vi "ep_Check One Trigger 1pt.vi"(6 "trig. local in":T1, 7 "prev. state in":i8, 8 "error in (no error)":errorcluster, 9 "data time stamp":timestamp, 10 "value in":dbl, 11 "trigger definition":T3) -> (0 "error out":errorcluster, 3 "triggers list":T2(array[cluster]), 4 "trig. local out":T1, 5 "state out":i8)   [LabVIEW 2011, in "NI_EP_Power Quality.lvlib"]
uses:
  <vilib>/addons/Electrical Power/PQ/NI_EP_Power Quality.lvlib
  <vilib>/addons/Electrical Power/PQ/Triggers/subVIs/ep_Trigger Definition.ctl
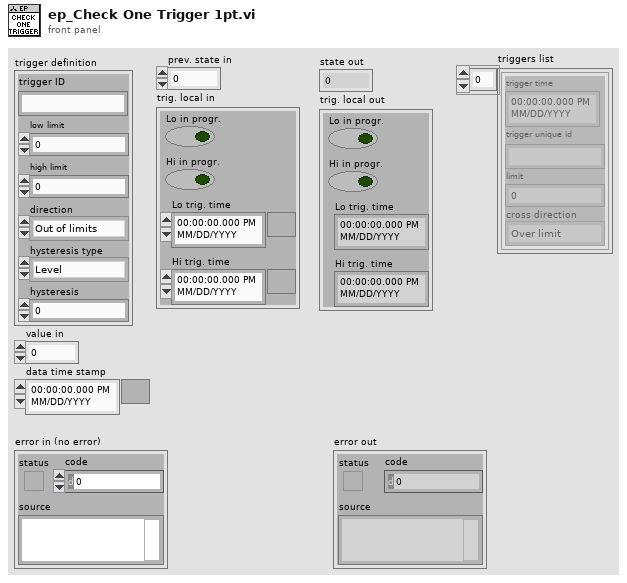
[diagram p1: front panel]
types:
  T1 = cluster{"Lo in progr.":bool, "Hi in progr.":bool, "Lo trig. time":timestamp, "Hi trig. time":timestamp}
  T2 = cluster{"trigger time":timestamp, "trigger unique id":string, "limit":dbl, "cross direction":enum16{"Over limit", "Below limit"}}[]
  T3 = typedef "NI_EP_Power Quality.lvlib/ep_Trigger Definition.ctl" = cluster{"trigger ID":string, "low limit":dbl, "high limit":dbl, "direction":enum16{"Out of limits", "Back to limits", "Both"}, "hysteresis type":enum16{"Level", "Time"}, "hysteresis":dbl}
  T4 = enum16{"Out of limits", "Back to limits", "Both"}
  T5 = cluster{"trigger time":timestamp, "trigger unique id":string, "limit":dbl, "cross direction":enum16{"Over limit", "Below limit"}}
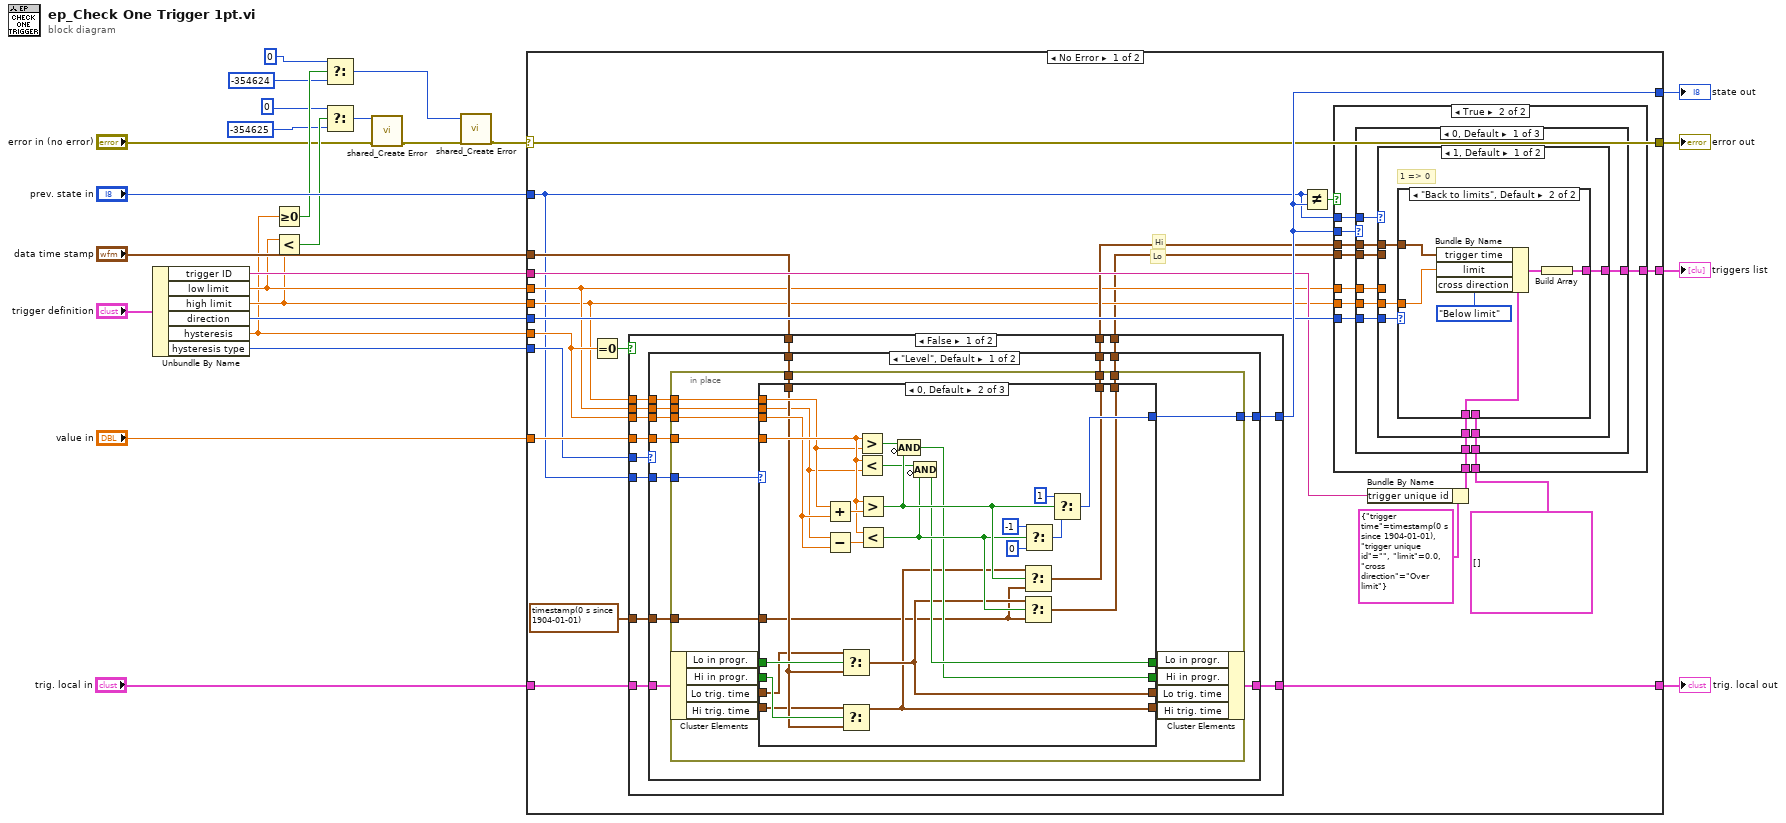
[diagram p0: block diagram]
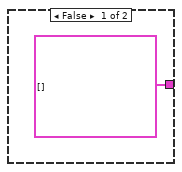
[diagram p2: hidden frame]
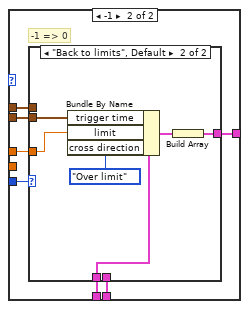
[diagram p4: hidden frame]
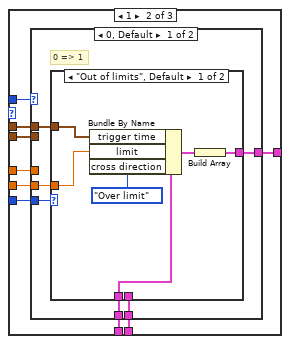
[diagram p6: hidden frame]
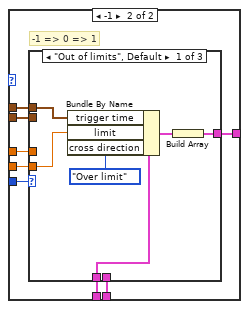
[diagram p8: hidden frame]
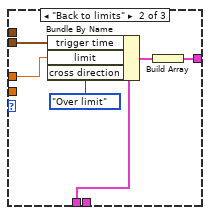
[diagram p9: hidden frame]
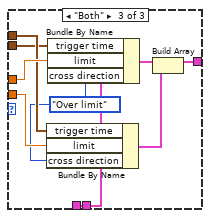
[diagram p10: hidden frame]
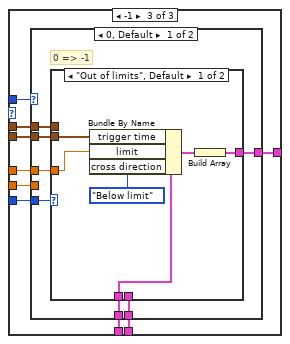
[diagram p11: hidden frame]
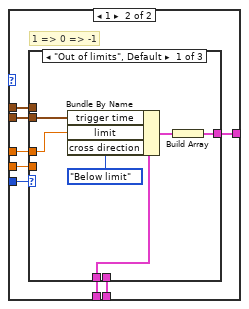
[diagram p13: hidden frame]
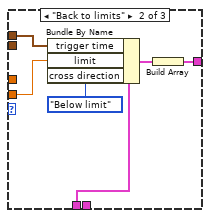
[diagram p14: hidden frame]
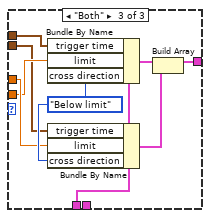
[diagram p15: hidden frame]
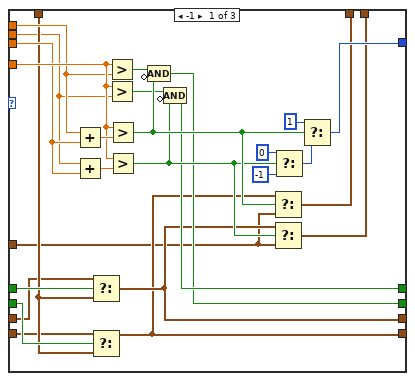
[diagram p16: hidden frame]
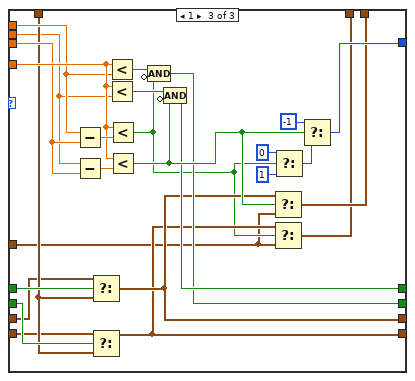
[diagram p17: hidden frame]
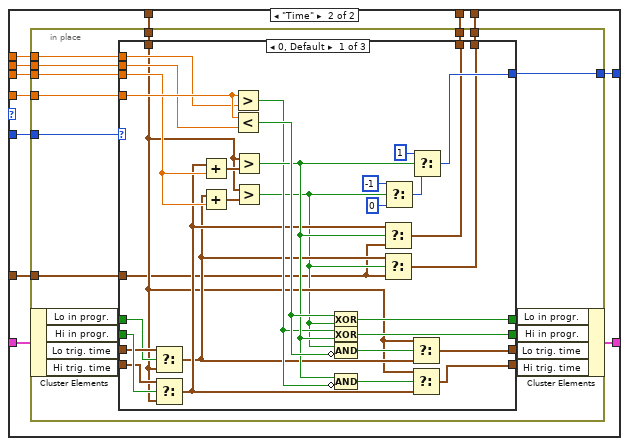
[diagram p18: hidden frame]
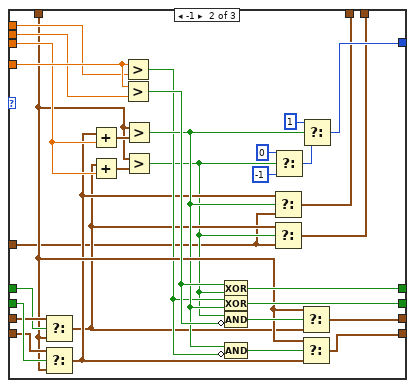
[diagram p19: hidden frame]
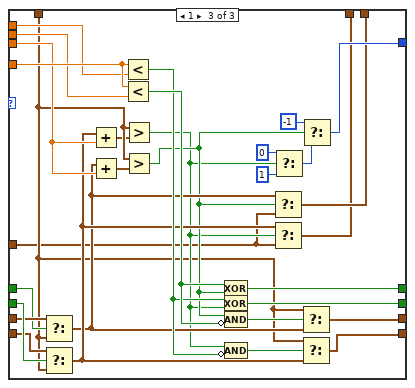
[diagram p20: hidden frame]
diagram:
  n1 = Unbundle By Name("trigger definition") -> ("trigger ID"=w22:string, "low limit"=w15:dbl, "high limit"=w14:dbl, "direction"=w23:T4, "hysteresis"=w11:dbl, "hysteresis type"=w16:enum16{"Level", "Time"})
  n2 = Greater Or Equal To 0?(x=w11) -> (x >= 0?=w10:bool)
  n3 = Less?(x=w15, y=w14) -> (x < y?=w13:bool)
  n4 = Select(t=0 ("error code (0)"), s=w10, f=-354624 ("error code (0)")) -> (s? t:f=w5:i32)
  n5 = Select(t=0 ("error code (0)"), s=w13, f=-354625 ("error code (0)")) -> (s? t:f=w1:i32)
  n6 = call <vilib>:"shared_Create Error.vi"("error in (no error)"="error in (no error)", "error code (0)"=w1) -> ("error out"=w3:errorcluster)  [unwired: 9 in]
  n7 = call <vilib>:"shared_Create Error.vi"("error in (no error)"=w3, "error code (0)"=w5) -> ("error out"=w6:errorcluster)  [unwired: 9 in]
  n8 = case shown="No Error" w6 {
    selector: w6 -> [w29 w460]
    tunnel: "value in" -> [w47 _]
    tunnel: [w45 _] -> w24
    tunnel: w23 -> [w44 _]
    tunnel: w22 -> [w42 _]
    tunnel: [w40 _] -> w21
    tunnel: w11 -> [w38 _]
    tunnel: [w37 _] -> w20
    tunnel: "prev. state in" -> [w28 _]
    tunnel: "data time stamp" -> [w36 _]
    tunnel: "trig. local in" -> [w34 _]
    tunnel: w16 -> [w32 _]
    tunnel: w15 -> [w31 _]
    tunnel: w14 -> [w30 _]
    tunnel: [w29 w460] -> w12
    frame No Error {
      # "Lo"
      # "Hi"
      n9 = Equal To 0?(x=w38) -> (x = 0?=w48:bool)
      n10 = case shown="False" w48 {
        tunnel: w47 -> [w203 w448]
        tunnel: w30 -> [w206 w450]
        tunnel: w31 -> [w205 w449]
        tunnel: [w210 w451] -> w45
        tunnel: w32 -> [w211 _]
        tunnel: w38 -> [w204 _]
        tunnel: w34 -> [w209 w447]
        tunnel: [w208 w447] -> w37
        tunnel: w28 -> [w207 _]
        tunnel: w36 -> [w202 w446]
        tunnel: [w201 w446] -> w35
        tunnel: timestamp(0 s since 1904-01-01) ("f") -> [w200 _]
        tunnel: [w199 w446] -> w27
        frame False {
          n11 = case shown="\"Level\", Default" w211 {
            tunnel: [w213 w330] -> w210
            tunnel: w209 -> [w222 w334]
            tunnel: [w221 w324] -> w208
            tunnel: w207 -> [w215 w329]
            tunnel: w206 -> [w219 w325]
            tunnel: w205 -> [w218 w326]
            tunnel: w204 -> [w217 w327]
            tunnel: w203 -> [w216 w328]
            tunnel: w202 -> [w220 w332]
            tunnel: [w214 w331] -> w201
            tunnel: w200 -> [w223 w333]
            tunnel: [w212 w323] -> w199
            frame "Level", Default {
              n12 = in-place {
                in-place-border: w223 -> [w233]
                in-place-border: w220 -> [w232]
                in-place-border: w219 -> [w231]
                in-place-border: w218 -> [w230]
                in-place-border: w217 -> [w229]
                in-place-border: w216 -> [w228]
                in-place-border: w215 -> [w227]
                in-place-border: [w226] -> w214
                in-place-border: [w225] -> w213
                in-place-border: [w224] -> w212
                n13 = in-place-cluster #1(w222) -> ("Lo in progr."=w241:bool, "Hi in progr."=w240:bool, "Lo trig. time"=w239:timestamp, "Hi trig. time"=w238:timestamp)
                n14 = case shown="0, Default" w227 {
                  tunnel: w241 -> [w253 w280 w310]
                  tunnel: w240 -> [w252 w279 w309]
                  tunnel: w239 -> [w249 w276 w304]
                  tunnel: w238 -> [w248 w275 w305]
                  tunnel: w231 -> [w266 w293 w320]
                  tunnel: w230 -> [w250 w277 w307]
                  tunnel: w229 -> [w265 w292 w319]
                  tunnel: w228 -> [w267 w294 w321]
                  tunnel: w232 -> [w251 w278 w308]
                  tunnel: [w259 w286 w313] -> w225
                  tunnel: [w258 w285 w296] -> w226
                  tunnel: w233 -> [w242 w270 w297]
                  tunnel: [w247 w274 w303] -> w237
                  tunnel: [w246 w273 w302] -> w236
                  tunnel: [w245 w272 w301] -> w235
                  tunnel: [w244 w271 w300] -> w234
                  tunnel: [w243 w269 w298] -> w224
                  frame -1 {
                    n15 = Add(x=w266, y=w265) -> (x+y=w268:dbl)
                    n16 = Add(x=w250, y=w265) -> (x+y=w264:dbl)
                    n17 = Select(t=w249, s=w253, f=w251) -> (s? t:f=w245:timestamp)
                    n18 = Select(t=w248, s=w252, f=w251) -> (s? t:f=w244:timestamp)
                    n19 = Greater?(x=w267, y=w266) -> (0:w257:bool)
                    n20 = Greater?(x=w267, y=w250) -> (0:w255:bool)
                    n21 = Greater?(x=w267, y=w268) -> (0:w256:bool)
                    n22 = Greater?(x=w267, y=w264) -> (0:w254:bool)
                    n23 = Compound Arithmetic op=AND(w257, invert w256) -> (w246:bool)
                    n24 = Compound Arithmetic op=AND(w255, invert w254) -> (w247:bool)
                    n25 = Select(t=w244, s=w256, f=w242) -> (s? t:f=w258:timestamp)
                    n26 = Select(t=w245, s=w254, f=w242) -> (s? t:f=w243:timestamp)
                    n27 = Select(t=i8 0 ("f"), s=w254, f=i8 -1) -> (s? t:f=w261:i8)
                    n28 = Select(t=i8 1 ("f"), s=w256, f=w261) -> (s? t:f=w259:i8)
                  }
                  frame 0, Default {
                    n29 = Add(x=w293, y=w292) -> (x+y=w295:dbl)
                    n30 = Subtract(x=w277, y=w292) -> (x-y=w291:dbl)
                    n31 = Select(t=w276, s=w280, f=w278) -> (s? t:f=w272:timestamp)
                    n32 = Select(t=w275, s=w279, f=w278) -> (s? t:f=w271:timestamp)
                    n33 = Greater?(x=w294, y=w293) -> (0:w284:bool)
                    n34 = Less?(x=w294, y=w277) -> (x < y?=w282:bool)
                    n35 = Greater?(x=w294, y=w295) -> (0:w283:bool)
                    n36 = Less?(x=w294, y=w291) -> (x < y?=w281:bool)
                    n37 = Compound Arithmetic op=AND(w284, invert w283) -> (w273:bool)
                    n38 = Compound Arithmetic op=AND(w282, invert w281) -> (w274:bool)
                    n39 = Select(t=w271, s=w283, f=w270) -> (s? t:f=w285:timestamp)
                    n40 = Select(t=w272, s=w281, f=w270) -> (s? t:f=w269:timestamp)
                    n41 = Select(t=i8 -1 ("f"), s=w281, f=i8 0) -> (s? t:f=w288:i8)
                    n42 = Select(t=i8 1 ("f"), s=w283, f=w288) -> (s? t:f=w286:i8)
                  }
                  frame 1 {
                    n43 = Subtract(x=w320, y=w319) -> (x-y=w322:dbl)
                    n44 = Subtract(x=w307, y=w319) -> (x-y=w318:dbl)
                    n45 = Select(t=w304, s=w310, f=w308) -> (s? t:f=w301:timestamp)
                    n46 = Select(t=w305, s=w309, f=w308) -> (s? t:f=w300:timestamp)
                    n47 = Less?(x=w321, y=w320) -> (x < y?=w312:bool)
                    n48 = Less?(x=w321, y=w307) -> (x < y?=w311:bool)
                    n49 = Less?(x=w321, y=w322) -> (x < y?=w299:bool)
                    n50 = Less?(x=w321, y=w318) -> (x < y?=w306:bool)
                    n51 = Compound Arithmetic op=AND(w312, invert w299) -> (w302:bool)
                    n52 = Compound Arithmetic op=AND(w311, invert w306) -> (w303:bool)
                    n53 = Select(t=w301, s=w306, f=w297) -> (s? t:f=w298:timestamp)
                    n54 = Select(t=w300, s=w299, f=w297) -> (s? t:f=w296:timestamp)
                    n55 = Select(t=i8 0 ("f"), s=w299, f=i8 1) -> (s? t:f=w315:i8)
                    n56 = Select(t=i8 -1 ("f"), s=w306, f=w315) -> (s? t:f=w313:i8)
                  }
                }
                n57 = in-place-cluster #1("Lo in progr."=w237, "Hi in progr."=w236, "Lo trig. time"=w235, "Hi trig. time"=w234) -> (w221:T1)
              }
            }
            frame "Time" {
              n58 = in-place {
                in-place-border: w333 -> [w344]
                in-place-border: w332 -> [w343]
                in-place-border: [w342] -> w331
                in-place-border: [w341] -> w330
                in-place-border: w329 -> [w340]
                in-place-border: w328 -> [w339]
                in-place-border: w327 -> [w338]
                in-place-border: w326 -> [w337]
                in-place-border: w325 -> [w336]
                in-place-border: [w335] -> w323
                n59 = in-place-cluster #2(w334) -> ("Lo in progr."=w352:bool, "Hi in progr."=w351:bool, "Lo trig. time"=w350:timestamp, "Hi trig. time"=w349:timestamp)
                n60 = case shown="0, Default" w340 {
                  tunnel: w352 -> [w368 w398 w431]
                  tunnel: w351 -> [w374 w404 w437]
                  tunnel: w350 -> [w372 w402 w435]
                  tunnel: w349 -> [w371 w401 w434]
                  tunnel: w336 -> [w381 w412 w444]
                  tunnel: w337 -> [w373 w403 w436]
                  tunnel: w338 -> [w370 w400 w433]
                  tunnel: w339 -> [w382 w413 w445]
                  tunnel: w343 -> [w357 w391 w419]
                  tunnel: [w376 w406 w438] -> w341
                  tunnel: [w375 w405 w415] -> w342
                  tunnel: w344 -> [w354 w385 w417]
                  tunnel: [w365 w395 w428] -> w348
                  tunnel: [w369 w399 w432] -> w347
                  tunnel: [w366 w396 w429] -> w346
                  tunnel: [w362 w392 w425] -> w345
                  tunnel: [w353 w384 w416] -> w335
                  frame 0, Default {
                    n61 = Select(t=w372, s=w368, f=w357) -> (s? t:f=w358:timestamp)
                    n62 = Select(t=w371, s=w374, f=w357) -> (s? t:f=w359:timestamp)
                    n63 = Add(x=w359, y=w370) -> (x+y=w383:timestamp)
                    n64 = Add(x=w358, y=w370) -> (x+y=w356:timestamp)
                    n65 = Greater?(x=w382, y=w381) -> (0:w360:bool)
                    n66 = Less?(x=w382, y=w373) -> (x < y?=w367:bool)
                    n67 = Greater?(x=w357, y=w383) -> (0:w361:bool)
                    n68 = Greater?(x=w357, y=w356) -> (0:w355:bool)
                    n69 = Exclusive Or(1:w355, 2:w367) -> (0:w365:bool)
                    n70 = Exclusive Or(1:w361, 2:w360) -> (0:w369:bool)
                    n71 = Compound Arithmetic op=AND(w355, invert w367) -> (w364:bool)
                    n72 = Compound Arithmetic op=AND(w361, invert w360) -> (w363:bool)
                    n73 = Select(t=w359, s=w361, f=w354) -> (s? t:f=w375:timestamp)
                    n74 = Select(t=w358, s=w355, f=w354) -> (s? t:f=w353:timestamp)
                    n75 = Select(t=i8 -1 ("f"), s=w355, f=i8 0) -> (s? t:f=w378:i8)
                    n76 = Select(t=w357, s=w364, f=w358) -> (s? t:f=w366:timestamp)
                    n77 = Select(t=w357, s=w363, f=w359) -> (s? t:f=w362:timestamp)
                    n78 = Select(t=i8 1 ("f"), s=w361, f=w378) -> (s? t:f=w376:i8)
                  }
                  frame -1 {
                    n79 = Select(t=w402, s=w398, f=w391) -> (s? t:f=w387:timestamp)
                    n80 = Select(t=w401, s=w404, f=w391) -> (s? t:f=w388:timestamp)
                    n81 = Add(x=w388, y=w400) -> (x+y=w414:timestamp)
                    n82 = Add(x=w387, y=w400) -> (x+y=w411:timestamp)
                    n83 = Greater?(x=w413, y=w412) -> (0:w389:bool)
                    n84 = Greater?(x=w413, y=w403) -> (0:w397:bool)
                    n85 = Greater?(x=w391, y=w414) -> (0:w390:bool)
                    n86 = Greater?(x=w391, y=w411) -> (0:w386:bool)
                    n87 = Exclusive Or(1:w386, 2:w397) -> (0:w395:bool)
                    n88 = Exclusive Or(1:w390, 2:w389) -> (0:w399:bool)
                    n89 = Compound Arithmetic op=AND(w386, invert w397) -> (w394:bool)
                    n90 = Compound Arithmetic op=AND(w390, invert w389) -> (w393:bool)
                    n91 = Select(t=w388, s=w390, f=w385) -> (s? t:f=w405:timestamp)
                    n92 = Select(t=w387, s=w386, f=w385) -> (s? t:f=w384:timestamp)
                    n93 = Select(t=i8 0 ("f"), s=w386, f=i8 -1) -> (s? t:f=w408:i8)
                    n94 = Select(t=w391, s=w394, f=w387) -> (s? t:f=w396:timestamp)
                    n95 = Select(t=w391, s=w393, f=w388) -> (s? t:f=w392:timestamp)
                    n96 = Select(t=i8 1 ("f"), s=w390, f=w408) -> (s? t:f=w406:i8)
                  }
                  frame 1 {
                    n97 = Select(t=w435, s=w431, f=w419) -> (s? t:f=w422:timestamp)
                    n98 = Select(t=w434, s=w437, f=w419) -> (s? t:f=w423:timestamp)
                    n99 = Add(x=w423, y=w433) -> (x+y=w418:timestamp)
                    n100 = Add(x=w422, y=w433) -> (x+y=w443:timestamp)
                    n101 = Less?(x=w445, y=w444) -> (x < y?=w424:bool)
                    n102 = Less?(x=w445, y=w436) -> (x < y?=w430:bool)
                    n103 = Greater?(x=w419, y=w418) -> (0:w420:bool)
                    n104 = Greater?(x=w419, y=w443) -> (0:w421:bool)
                    n105 = Exclusive Or(1:w421, 2:w430) -> (0:w428:bool)
                    n106 = Exclusive Or(1:w420, 2:w424) -> (0:w432:bool)
                    n107 = Compound Arithmetic op=AND(w421, invert w430) -> (w427:bool)
                    n108 = Compound Arithmetic op=AND(w420, invert w424) -> (w426:bool)
                    n109 = Select(t=w422, s=w421, f=w417) -> (s? t:f=w416:timestamp)
                    n110 = Select(t=w423, s=w420, f=w417) -> (s? t:f=w415:timestamp)
                    n111 = Select(t=i8 0 ("f"), s=w420, f=i8 1) -> (s? t:f=w440:i8)
                    n112 = Select(t=w419, s=w427, f=w422) -> (s? t:f=w429:timestamp)
                    n113 = Select(t=w419, s=w426, f=w423) -> (s? t:f=w425:timestamp)
                    n114 = Select(t=i8 -1 ("f"), s=w421, f=w440) -> (s? t:f=w438:i8)
                  }
                }
                n115 = in-place-cluster #2("Lo in progr."=w348, "Hi in progr."=w347, "Lo trig. time"=w346, "Hi trig. time"=w345) -> (w324:T1)
              }
            }
          }
        }
        frame True {
          n116 = In Range and Coerce(upper limit=w450, x=w448, lower limit=w449) -> (In Range?=w452:bool)  [unwired: 1 out]
          n117 = case shown="False" w452 {
            tunnel: [w453 i8 0 ("f")] -> w451
            tunnel: w450 -> [w457 _]
            tunnel: w448 -> [w458 _]
            frame False {
              n118 = Greater?(x=w458, y=w457) -> (0:w454:bool)
              n119 = Select(t=i8 1, s=w454, f=i8 -1) -> (s? t:f=w453:i8)
            }
            frame True {
            }
          }
        }
      }
      n120 = Not Equal?(x=w28, y=w45) -> (x != y?=w46:bool)
      n121 = Bundle By Name(cluster=T5 {"trigger time"=timestamp(0 s since 1904-01-01), "trigger unique id"="", "limit"=0.0, "cross direction"=enum."Over limit"} ("trigger"), "trigger unique id"=w42) -> (w41:T5)
      n122 = case shown="True" w46 {
        tunnel: w28 -> [_ w58]
        tunnel: w45 -> [_ w59]
        tunnel: w31 -> [_ w53]
        tunnel: w30 -> [_ w57]
        tunnel: w44 -> [_ w55]
        tunnel: w35 -> [_ w54]
        tunnel: w41 -> [_ w56]
        tunnel: [T2 [] w52] -> w40
        tunnel: T2 [] -> [_ w51]
        tunnel: w27 -> [_ w50]
        frame False {
        }
        frame True {
          n123 = case shown="0, Default" w59 {
            tunnel: w58 -> [w68 w104 w155]
            tunnel: w57 -> [w67 w103 w154]
            tunnel: w56 -> [w66 w102 w153]
            tunnel: w55 -> [w65 w101 w152]
            tunnel: w54 -> [w64 w100 w151]
            tunnel: w53 -> [w63 w99 w150]
            tunnel: [w62 w98 w149] -> w52
            tunnel: w51 -> [w61 w97 w148]
            tunnel: w50 -> [w60 w96 w147]
            frame 0, Default {
              n124 = case shown="1, Default" w68 {
                tunnel: w67 -> [w71 _]
                tunnel: w66 -> [w73 w87]
                tunnel: w65 -> [w74 w88]
                tunnel: w64 -> [w72 w86]
                tunnel: w63 -> [_ w83]
                tunnel: [w70 w85] -> w62
                tunnel: w61 -> [w69 w84]
                tunnel: w60 -> [_ w82]
                frame 1, Default {
                  # "1 => 0"
                  n125 = case shown="\"Back to limits\", Default" w74 {
                    tunnel: w73 -> [_ w81]
                    tunnel: w72 -> [_ w76]
                    tunnel: w71 -> [_ w80]
                    tunnel: [w75 w77] -> w70
                    tunnel: w69 -> [w75 _]
                    frame "Out of limits" {
                    }
                    frame "Back to limits", Default {
                      n126 = Bundle By Name(cluster=w81, "trigger time"=w76, "limit"=w80, "cross direction"=enum16{"Over limit", "Below limit"}."Below limit") -> (w78:T5)
                      n127 = Build Array(w78) -> (w77:T2)
                    }
                  }
                }
                frame -1 {
                  # "-1 => 0"
                  n128 = case shown="\"Back to limits\", Default" w88 {
                    tunnel: w87 -> [_ w95]
                    tunnel: w86 -> [_ _]
                    tunnel: [w89 w92] -> w85
                    tunnel: w84 -> [w89 _]
                    tunnel: w83 -> [_ w91]
                    tunnel: w82 -> [_ w90]
                    frame "Out of limits" {
                    }
                    frame "Back to limits", Default {
                      n129 = Bundle By Name(cluster=w95, "trigger time"=w90, "limit"=w91, "cross direction"=enum16{"Over limit", "Below limit"}."Over limit") -> (w93:T5)
                      n130 = Build Array(w93) -> (w92:T2)
                    }
                  }
                }
              }
            }
            frame 1 {
              n131 = case shown="0, Default" w104 {
                tunnel: w103 -> [w107 w122]
                tunnel: w102 -> [w109 w124]
                tunnel: w101 -> [w110 w125]
                tunnel: w100 -> [w108 w123]
                tunnel: w99 -> [_ w119]
                tunnel: [w106 w121] -> w98
                tunnel: w97 -> [w105 w120]
                tunnel: w96 -> [_ w118]
                frame 0, Default {
                  # "0 => 1"
                  n132 = case shown="\"Out of limits\", Default" w110 {
                    tunnel: w109 -> [w116 _]
                    tunnel: w108 -> [w115 _]
                    tunnel: w107 -> [w114 _]
                    tunnel: [w111 w117] -> w106
                    tunnel: w105 -> [_ w117]
                    frame "Out of limits", Default {
                      n133 = Bundle By Name(cluster=w116, "trigger time"=w115, "limit"=w114, "cross direction"=enum16{"Over limit", "Below limit"}."Over limit") -> (w112:T5)
                      n134 = Build Array(w112) -> (w111:T2)
                    }
                    frame "Back to limits" {
                    }
                  }
                }
                frame -1 {
                  # "-1 => 0 => 1"
                  n135 = case shown="\"Out of limits\", Default" w125 {
                    tunnel: w124 -> [w131 w137 w141]
                    tunnel: w123 -> [w130 _ w143]
                    tunnel: w122 -> [w126 _ w142]
                    tunnel: [w127 w134 w145] -> w121
                    tunnel: w120 -> [_ _ _]
                    tunnel: w119 -> [_ w133 w144]
                    tunnel: w118 -> [_ w132 w138]
                    frame "Out of limits", Default {
                      n136 = Bundle By Name(cluster=w131, "trigger time"=w130, "limit"=w126, "cross direction"=enum16{"Over limit", "Below limit"}."Over limit") -> (w128:T5)
                      n137 = Build Array(w128) -> (w127:T2)
                    }
                    frame "Back to limits" {
                      n138 = Bundle By Name(cluster=w137, "trigger time"=w132, "limit"=w133, "cross direction"=enum16{"Over limit", "Below limit"}."Over limit") -> (w135:T5)
                      n139 = Build Array(w135) -> (w134:T2)
                    }
                    frame "Both" {
                      w139 = enum16{"Over limit", "Below limit"}."Over limit" ("cross direction")
                      n140 = Bundle By Name(cluster=w141, "trigger time"=w143, "limit"=w142, "cross direction"=w139) -> (w140:T5)
                      n141 = Bundle By Name(cluster=w141, "trigger time"=w138, "limit"=w144, "cross direction"=w139) -> (w146:T5)
                      n142 = Build Array(w146, w140) -> (w145:T2)
                    }
                  }
                }
              }
            }
            frame -1 {
              n143 = case shown="0, Default" w155 {
                tunnel: w154 -> [_ w174]
                tunnel: w153 -> [w161 w176]
                tunnel: w152 -> [w162 w177]
                tunnel: w151 -> [w160 w175]
                tunnel: w150 -> [w157 w171]
                tunnel: [w159 w173] -> w149
                tunnel: w148 -> [w158 w172]
                tunnel: w147 -> [w156 w170]
                frame 0, Default {
                  # "0 => -1"
                  n144 = case shown="\"Out of limits\", Default" w162 {
                    tunnel: w161 -> [w168 _]
                    tunnel: w160 -> [_ _]
                    tunnel: [w165 w169] -> w159
                    tunnel: w158 -> [_ w169]
                    tunnel: w157 -> [w164 _]
                    tunnel: w156 -> [w163 _]
                    frame "Out of limits", Default {
                      n145 = Bundle By Name(cluster=w168, "trigger time"=w163, "limit"=w164, "cross direction"=enum16{"Over limit", "Below limit"}."Below limit") -> (w166:T5)
                      n146 = Build Array(w166) -> (w165:T2)
                    }
                    frame "Back to limits" {
                    }
                  }
                }
                frame 1 {
                  # "1 => 0 => -1"
                  n147 = case shown="\"Out of limits\", Default" w177 {
                    tunnel: w176 -> [w183 w189 w195]
                    tunnel: w175 -> [_ w188 w196]
                    tunnel: w174 -> [_ w184 w191]
                    tunnel: [w180 w185 w197] -> w173
                    tunnel: w172 -> [_ _ _]
                    tunnel: w171 -> [w179 _ w192]
                    tunnel: w170 -> [w178 _ w190]
                    frame "Out of limits", Default {
                      n148 = Bundle By Name(cluster=w183, "trigger time"=w178, "limit"=w179, "cross direction"=enum16{"Over limit", "Below limit"}."Below limit") -> (w181:T5)
                      n149 = Build Array(w181) -> (w180:T2)
                    }
                    frame "Back to limits" {
                      n150 = Bundle By Name(cluster=w189, "trigger time"=w188, "limit"=w184, "cross direction"=enum16{"Over limit", "Below limit"}."Below limit") -> (w186:T5)
                      n151 = Build Array(w186) -> (w185:T2)
                    }
                    frame "Both" {
                      w193 = enum16{"Over limit", "Below limit"}."Below limit" ("cross direction")
                      n152 = Bundle By Name(cluster=w195, "trigger time"=w196, "limit"=w191, "cross direction"=w193) -> (w198:T5)
                      n153 = Bundle By Name(cluster=w195, "trigger time"=w190, "limit"=w192, "cross direction"=w193) -> (w194:T5)
                      n154 = Build Array(w198, w194) -> (w197:T2)
                    }
                  }
                }
              }
            }
          }
        }
      }
    }
    frame Error {
    }
  }
  "state out" <- w24
  "triggers list" <- w21
  "trig. local out" <- w20
  "error out" <- w12
